vi "2283_calibrarElevador.vi"(0 "input cluster":T2, 1 "Potenciometro linear":dbl(knob) scale=-1.0..1.0) -> (2 "Output elevador":dbl, 3 "Altura":dbl, 4 "Gripp output":bool, 5 "Cuernitos":bool)   [LabVIEW 2014]
uses:
  2283_Outputs autonomo.vi
  <vilib>/addons/control/pid/pid.llb/PID (DBL).vi
  <vilib>/addons/control/pid/NI_PID_pid.lvlib
panel:
  in  "x":dbl=50.0 format="%#_13g"
  in  "PID gains":T1={"proportional gain (Kc)"=0.035, "integral time (Ti, min)"=0.008, "derivative time (Td, min)"=0.0}
  in  "Nivel Cargar":dbl=60.0 format="%#_13g"
  in  "Nivel 1 Caja":dbl=225.0 format="%#_13g"
  in  "Nivel 2 Cajas":dbl=385.0 format="%#_13g"
  in  "Nivel 3 Cajas":dbl=560.0 format="%#_13g"
  in  "Dejar":dbl=530.0 format="%#_13g"
  in  "Nivel Step":dbl=165.0 format="%#_13g"
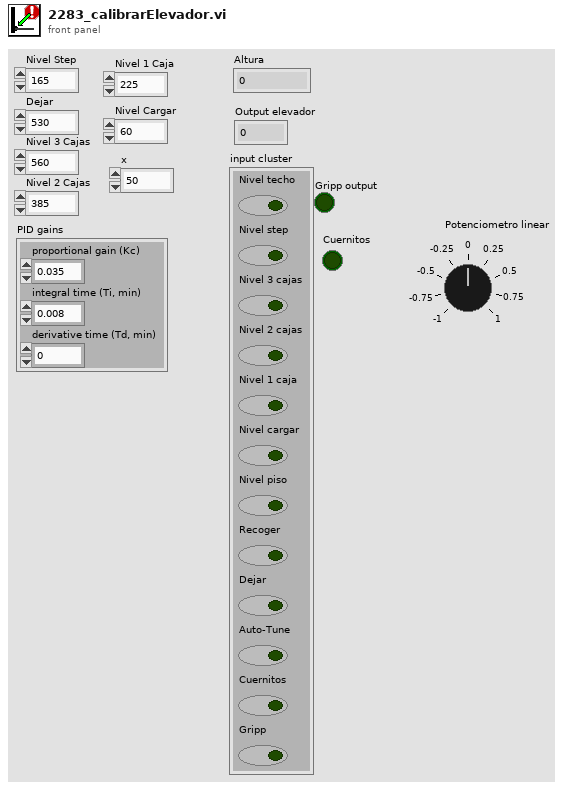
[diagram p1: front panel]
types:
  T1 = cluster{"proportional gain (Kc)":dbl, "integral time (Ti, min)":dbl, "derivative time (Td, min)":dbl}
  T2 = cluster{"Nivel techo":bool, "Nivel step":bool, "Nivel 3 cajas":bool, "Nivel 2 cajas":bool, "Nivel 1 caja":bool, "Nivel cargar":bool, "Nivel piso":bool, "Recoger":bool, "Dejar":bool, "Auto-Tune":bool, "Cuernitos":bool, "Gripp":bool}
  T3 = enum16{"NA", "Nivel cargar", "Nivel Techo", "Nivel step", "Nivel 3 cajas", "Nivel 2 cajas", "Nivel 1 caja", "Nivel Piso"}
  T4 = cluster{"Agarrar caja":bool, "Rotate":dbl, "Dejar caja":bool, "Activar moonwalk":bool, "Alejarse de la caja":bool, "PID LIdar":bool, "Aproach caja":bool, "Comer":bool, "Levante el bote":bool}
  T5 = typedef "WPI_SwitchDevRef.ctl" = cluster{"DevStatus":errorcluster, "DIO Channel":T6, "Controller":T7, "CntIndex":T8, "Normally Closed":bool}
  T6 = typedef "FPGA_DIOChannel.ctl" = enum8{"DIO 0", "DIO 1", "DIO 2", "DIO 3", "DIO 4", "DIO 5", "DIO 6", "DIO 7", "DIO 8", "DIO 9", "DIO MXP 0", "DIO MXP 1", "DIO MXP 2", "DIO MXP 3", "DIO MXP 4", "DIO MXP 5", "DIO MXP 6", "DIO MXP 7", "DIO MXP 8", "DIO MXP 9", "DIO MXP 10", "DIO MXP 11", "DIO MXP 12", "DIO MXP 13", "DIO MXP 14", "DIO MXP 15", "Invalid"}
  T7 = typedef "FPGA_TypedefDigitalModule.ctl" = enum16{"Controller 1"}
  T8 = typedef "FPGA_CounterCtrSystemIndex.ctl" = enum8{"Ctr 0", "Ctr 1", "Ctr 2", "Ctr 3", "Ctr 4", "Ctr 5", "Ctr 6", "Ctr 7", "Invalid"}
  T9 = typedef "WPI_EncoderDevRef.ctl" = cluster{"DevStatus":errorcluster, "EncoderIndex":T10, "CounterIndex":T8, "DistancePerCount":dbl, "Decoding Type":T11}
  T10 = typedef "FPGA_EncoderIdx.ctl" = enum8{"Enc 0", "Enc 1", "Enc 2", "Enc 3", "Enc 4", "Enc 5", "Enc 6", "Enc 7", "Invalid"}
  T11 = typedef "WPI_EncoderType.ctl" = enum16{"1x", "2x", "4x"}
  T12 = cluster{"Nivel techo":dbl, "Nivel 3 cajas":dbl, "Nivel 2 cajas":dbl, "Nivel 1 caja":dbl, "Nivel step":dbl, "Nivel cargar":dbl}
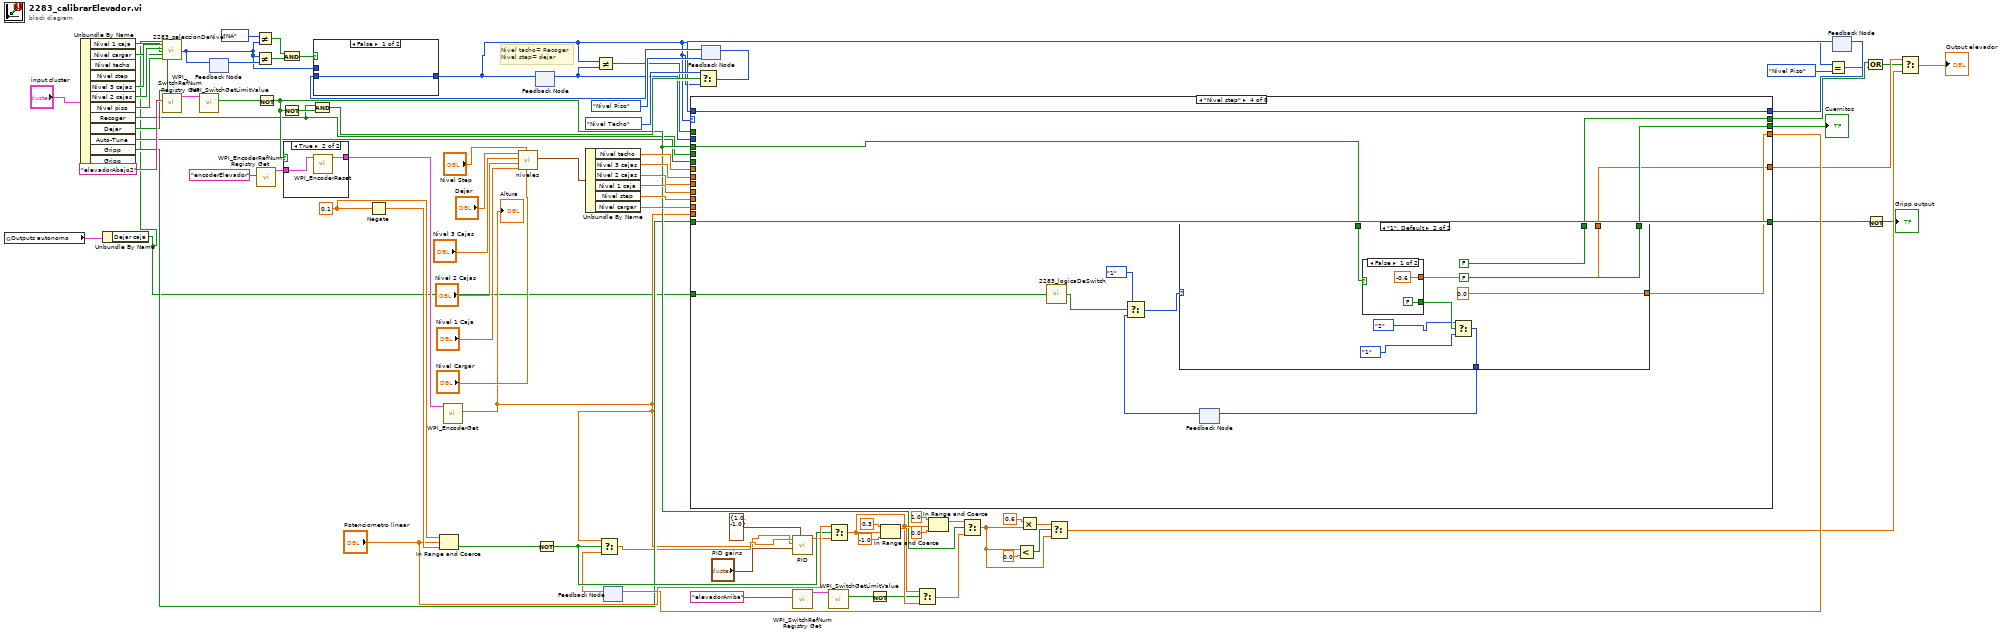
[diagram p0: block diagram]
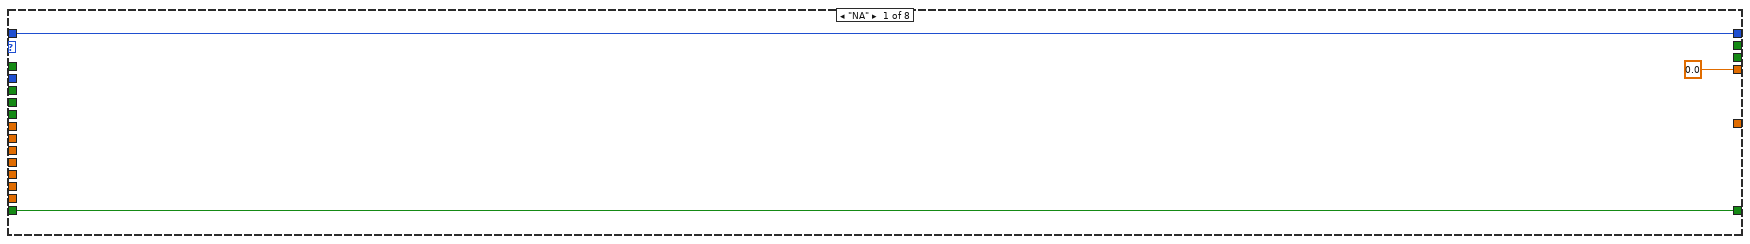
[diagram p2: hidden frame]
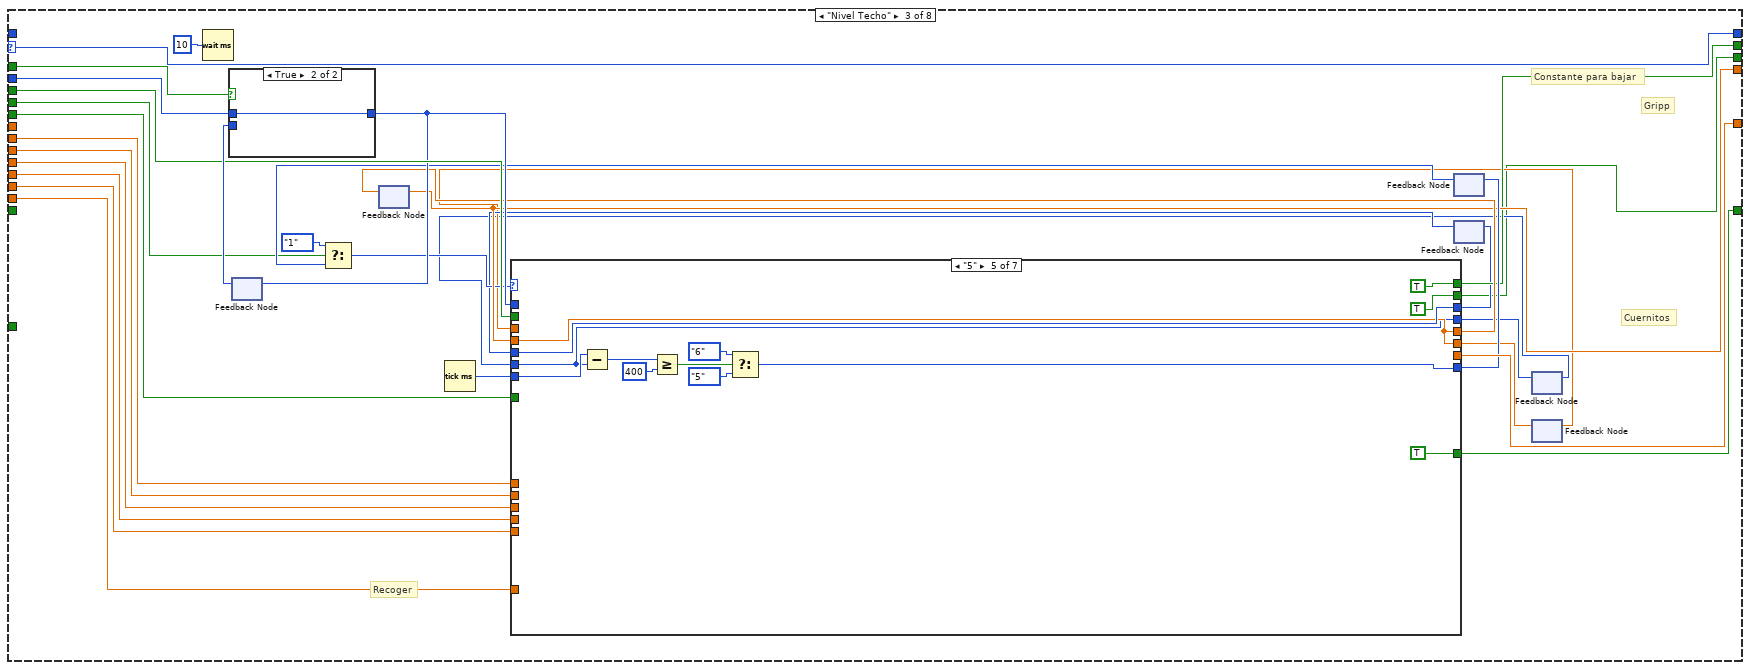
[diagram p4: hidden frame]
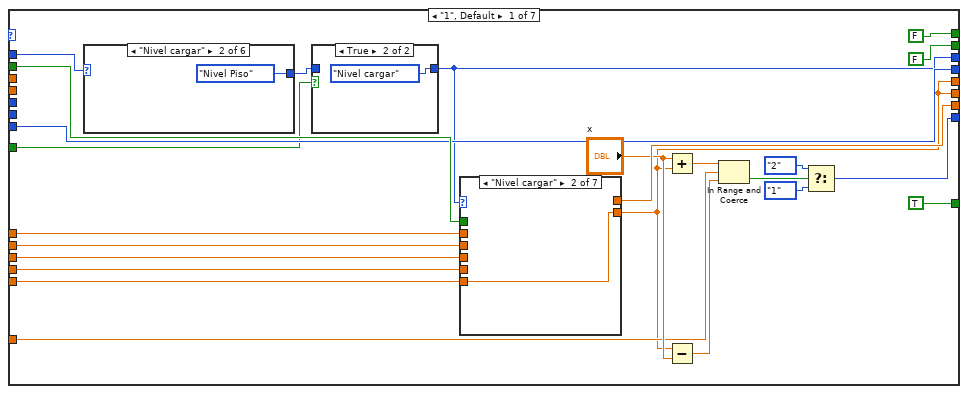
[diagram p5: hidden frame]
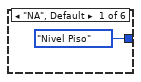
[diagram p7: hidden frame]
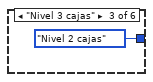
[diagram p8: hidden frame]
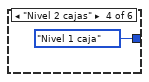
[diagram p9: hidden frame]
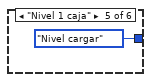
[diagram p10: hidden frame]
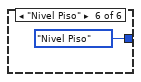
[diagram p11: hidden frame]
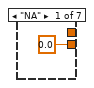
[diagram p12: hidden frame]
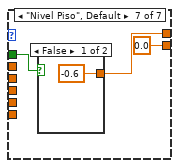
[diagram p17: hidden frame]
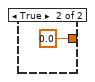
[diagram p18: hidden frame]
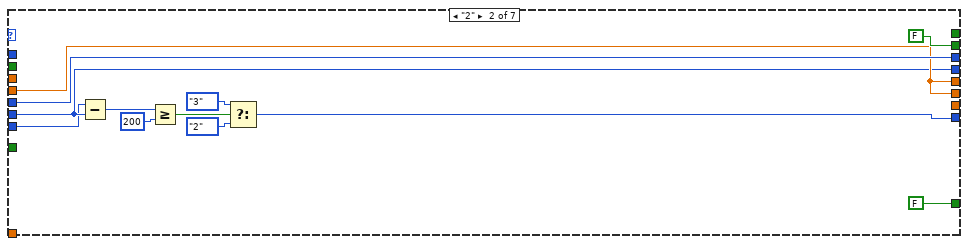
[diagram p19: hidden frame]
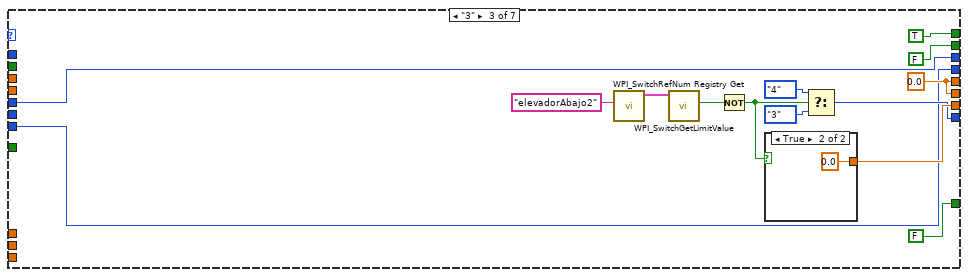
[diagram p20: hidden frame]
diagram:
  w81 = 0.1 ("upper limit")
  # "Nivel techo= Recoger\nNivel step= dejar"
  n1 = global read "2283_Outputs autonomo.vi" "Outputs autonomo"() -> (w2:T4)
  n2 = Unbundle By Name("input cluster") -> ("Nivel 1 caja"=w38:bool, "Nivel cargar"=w39:bool, "Nivel 3 cajas"=w40:bool, "Nivel 2 cajas"=w41:bool, "Nivel piso"=w42:bool, "Recoger"=w10:bool, "Dejar"=w11:bool, "Auto-Tune"=w5:bool, "Gripp"=w15:bool)  [unwired: 3 out]
  n3 = Unbundle By Name(w2) -> ("Dejar caja"=w1:bool)
  n4 = call "2283_seleccionDeNivel.vi"("Cargar"=w1, "Nivel 3 cajas"=w40, "Nivel 2 cajas"=w41, "Nivel 1 caja"=w38, "Nivel cargar"=w39, "Recoger"=w11, "Nivel piso"=w42) -> ("nivel"=w44:T3)  [unwired: 12 in]
  n5 = call <vilib>:"WPI_SwitchRefNum Registry Get.vi"("refnum name"="elevadorAbajo2") -> ("SwitchDevRef"=w83:T5)  [unwired: 9 in, 1 out]
  n6 = call <vilib>:"WPI_SwitchGetLimitValue.vi"("SwitchDevRef"=w83) -> ("Switch Pressed"=w20:bool)  [unwired: 8 in, 2 out]
  n7 = feedback-in #1(w44) -> ()
  n8 = feedback #1() -> (w65:T3)  [unwired: 1 in]
  n9 = Not Equal?(x=T3."NA" ("Enum"), y=w44) -> (x != y?=w66:bool)
  n10 = Not Equal?(x=w44, y=w65) -> (x != y?=w67:bool)
  n11 = call <vilib>:"WPI_EncoderRefNum Registry Get.vi"("refnum name"="encoderElevador") -> ("EncoderDevRef"=w86:T9)  [unwired: 9 in, 1 out]
  n12 = Not(x=w20) -> (.not. x?=w24:bool)
  n13 = And(x=w66, y=w67) -> (x .and. y?=w63:bool)
  n14 = Not(x=w24) -> (.not. x?=w28:bool)
  n15 = case shown="True" w24 {
    tunnel: w86 -> [w89 w91]
    tunnel: [w89 w90] -> w85
    frame False {
    }
    frame True {
      n16 = call <vilib>:"WPI_EncoderReset.vi"("EncoderDevRef"=w91) -> ("EncoderDevRef"=w90:T9)  [unwired: 9 in, 1 out]
    }
  }
  n17 = And(x=w10, y=w28) -> (x .and. y?=w54:bool)
  n18 = Negate(x=w81) -> (-x=w80:dbl)
  n19 = In Range and Coerce(upper limit=w81, x="Potenciometro linear", lower limit=w80) -> (In Range?=w79:bool)  [unwired: 1 out]
  n20 = call <vilib>:"WPI_EncoderGet.vi"("EncoderDevRef"=w85) -> ("Distance"=w3:dbl)  [unwired: 5 in, 5 out]
  "Altura" <- w3
  n21 = call "niveles.vi"("Nivel cargar"="Nivel Cargar", "Nivel step"="Nivel Step", "Nivel 1 caja"="Nivel 1 Caja", "Nivel 2 cajas"="Nivel 2 Cajas", "Nivel 3 cajas"="Nivel 3 Cajas", "Nivel techo"="Dejar") -> ("output cluster"=w51:T12)  [unwired: 5 in]
  n22 = feedback #2() -> (w6:T3)  [unwired: 1 in]
  n23 = Not(x=w79) -> (.not. x?=w77:bool)
  n24 = Unbundle By Name(w51) -> ("Nivel techo"=w60:dbl, "Nivel 3 cajas"=w58:dbl, "Nivel 2 cajas"=w57:dbl, "Nivel 1 caja"=w56:dbl, "Nivel step"=w59:dbl, "Nivel cargar"=w55:dbl)
  n25 = feedback #3() -> (w36:dbl)  [unwired: 1 in]
  n26 = Select(t=w3, s=w77, f=w36) -> (s? t:f=w4:dbl)
  n27 = feedback #4(T3."Nivel Piso" ("Enum")) -> (w62:T3)
  n28 = case shown="False" w63 {
    tunnel: w44 -> [_ w93]
    tunnel: [w92 w93] -> w8
    tunnel: w62 -> [w92 _]
    frame False {
    }
    frame True {
    }
  }
  n29 = feedback-in #2(w8) -> ()
  n30 = Not Equal?(x=w8, y=w6) -> (x != y?=w7:bool)
  n31 = Select(t=T3."Nivel Techo" ("Enum"), s=w54, f=w8) -> (s? t:f=w52:T3)
  n32 = feedback-in #4(w52) -> ()
  n33 = call-poly <vilib>:"PID.vi"("output range"=cluster{"output high":dbl, "output low":dbl} {"output high"=1.0, "output low"=-1.0}, "PID gains"="PID gains", "process variable"=w3, "setpoint"=w4) -> ("output"=w26:dbl)  [unwired: 6 in, 1 out]
  n34 = call <vilib>:"WPI_SwitchRefNum Registry Get.vi"("refnum name"="elevadorArriba") -> ("SwitchDevRef"=w87:T5)  [unwired: 9 in, 1 out]
  n35 = call <vilib>:"WPI_SwitchGetLimitValue.vi"("SwitchDevRef"=w87) -> ("Switch Pressed"=w74:bool)  [unwired: 8 in, 2 out]
  n36 = Select(t="Potenciometro linear", s=w77, f=w26) -> (s? t:f=w68:dbl)
  n37 = Not(x=w74) -> (.not. x?=w29:bool)
  n38 = In Range and Coerce(upper limit=0.3, x=w68, lower limit=-1.0) -> (coerced(x)=w75:dbl)  [unwired: 1 out]
  n39 = Select(t=w75, s=w29, f=w68) -> (s? t:f=w69:dbl)
  n40 = In Range and Coerce(upper limit=1.0, x=w68, lower limit=0.0) -> (coerced(x)=w71:dbl)  [unwired: 1 out]
  n41 = Select(t=w71, s=w24, f=w69) -> (s? t:f=w30:dbl)
  n42 = Less?(x=w30, y=0.0) -> (x < y?=w33:bool)
  n43 = Multiply(x=0.6, y=w30) -> (x*y=w31:dbl)
  n44 = Select(t=w31, s=w33, f=w30) -> (s? t:f=w21:dbl)
  n45 = Equal?(x=w8, y=T3."Nivel Piso" ("Enum")) -> (x = y?=w13:bool)
  n46 = feedback #5() -> (w35:T3)  [unwired: 1 in]
  n47 = case shown="\"Nivel step\"" w8 {
    selector: w8 -> [_ _ w130 _ _ _ _ _]
    tunnel: [0.0 ("upper limit") w99 w117 w287 w312 w315 w318 0.0 ("Nivel 1 caja")] -> w37
    tunnel: w60 -> [_ _ _ _ _ _ _ _]
    tunnel: w59 -> [_ _ w129 _ _ _ _ _]
    tunnel: w58 -> [_ _ w128 _ w312 _ _ _]
    tunnel: w57 -> [_ _ w127 _ _ w315 _ _]
    tunnel: w56 -> [_ _ w126 _ _ _ w318 _]
    tunnel: w55 -> [_ w99 w125 _ _ _ _ _]
    tunnel: [w95 w98 w130 w291 w311 w314 w317 w325] -> w18
    tunnel: w35 -> [w95 w98 _ w291 w311 w314 w317 w325]
    tunnel: w24 -> [_ _ w124 w285 _ _ _ w324]
    tunnel: [_ _ w122 w286 _ _ _ w322] -> w22
    tunnel: w15 -> [w94 w97 _ w290 w310 w313 w316 w321]
    tunnel: [w94 w97 w119 w290 w310 w313 w316 w321] -> w17
    tunnel: w3 -> [_ _ w121 _ _ _ _ _]
    tunnel: [_ _ w101 w288 _ _ _ FALSE] -> w16
    tunnel: [_ _ w113 w289 _ _ _ FALSE] -> w14
    tunnel: w6 -> [_ _ w110 _ _ _ _ _]
    tunnel: w10 -> [_ _ w103 _ _ _ _ _]
    tunnel: w7 -> [_ _ w102 _ _ _ _ _]
    tunnel: w5 -> [_ _ w100 _ _ _ _ _]
    tunnel: w1 -> [_ _ _ w281 _ _ _ _]
    frame "NA" {
    }
    frame "Nivel cargar" {
    }
    frame "Nivel Techo" {
      # "Cuernitos"
      # "Gripp"
      # "Constante para bajar"
      # "Recoger"
      n48 = Wait (ms)(milliseconds to wait=u32 10) -> ()  [unwired: 1 out]
      n49 = feedback #6() -> (w131:T3)  [unwired: 1 in]
      n50 = case shown="True" w102 {
        tunnel: w110 -> [_ w278]
        tunnel: [w277 w278] -> w123
        tunnel: w131 -> [w277 _]
        frame False {
        }
        frame True {
        }
      }
      n51 = feedback-in #6(w123) -> ()
      n52 = feedback #7() -> (w117:dbl)  [unwired: 1 in]
      n53 = Tick Count (ms)() -> (millisecond timer value=w104:u32)
      n54 = feedback #8() -> (w115:enum16{"1", "2", "3", "4", "5", "6", "7"})  [unwired: 1 in]
      n55 = Select(t=enum16{"1", "2", "3", "4", "5", "6", "7"}."1", s=w103, f=w115) -> (s? t:f=w114:enum16{"1", "2", "3", "4", "5", "6", "7"})
      n56 = feedback #9() -> (w111:T3)  [unwired: 1 in]
      n57 = feedback #10() -> (w105:u32)  [unwired: 1 in]
      n58 = feedback #11() -> (w107:dbl)  [unwired: 1 in]
      n59 = case shown="\"5\"" w114 {
        tunnel: w129 -> [w155 _ _ _ _ w248 _]
        tunnel: w128 -> [w154 _ _ _ _ w251 _]
        tunnel: w127 -> [w153 _ _ _ _ w250 _]
        tunnel: w126 -> [w152 _ _ _ _ w249 _]
        tunnel: w125 -> [w151 _ _ _ _ w247 _]
        tunnel: w124 -> [w150 _ _ _ _ w246 _]
        tunnel: w123 -> [w149 _ _ _ _ _ _]
        tunnel: [w132 w183 w189 w212 w227 w234 w275] -> w118
        tunnel: [w148 _ w200 _ _ w245 _] -> w122
        tunnel: w121 -> [w145 _ _ _ _ w235 _]
        tunnel: [w140 w181 w197 w209 w224 w236 enum16{"1", "2", "3", "4", "5", "6", "7"}."7"] -> w120
        tunnel: [TRUE FALSE FALSE TRUE TRUE TRUE TRUE] -> w119
        tunnel: w117 -> [_ w183 _ w212 w227 _ _]
        tunnel: [FALSE ("Cuernitos") FALSE ("Cuernitos") FALSE ("Cuernitos") FALSE ("Cuernitos") TRUE ("Cuernitos") FALSE ("Cuernitos") FALSE ("Cuernitos")] -> w101
        tunnel: [FALSE _ TRUE TRUE TRUE _ _] -> w113
        tunnel: [w134 w184 w190 w213 w228 w243 w273] -> w112
        tunnel: w111 -> [_ w184 w190 w213 w228 w243 w273]
        tunnel: [w132 w183 w189 w212 w227 w234 w275] -> w108
        tunnel: w107 -> [_ _ _ _ _ _ w275]
        tunnel: [w136 w176 w188 w204 w218 w233 w272] -> w106
        tunnel: w105 -> [_ w176 _ w204 w218 _ _]
        tunnel: w104 -> [w136 w175 w188 w205 w220 w233 w272]
        tunnel: w100 -> [w133 _ _ _ _ w229 _]
        frame "1", Default {
          n60 = case shown="\"Nivel cargar\"" w149 {
            tunnel: [T3."Nivel Piso" ("Enum") T3."Nivel Piso" ("Enum") T3."Nivel 2 cajas" ("Enum") T3."Nivel 1 caja" ("Enum") T3."Nivel cargar" ("Enum") T3."Nivel Piso" ("Enum")] -> w135
            frame "NA", Default {
            }
            frame "Nivel cargar" {
            }
            frame "Nivel 3 cajas" {
            }
            frame "Nivel 2 cajas" {
            }
            frame "Nivel 1 caja" {
            }
            frame "Nivel Piso" {
            }
          }
          n61 = case shown="True" w133 {
            tunnel: w135 -> [w156 _]
            tunnel: [w156 T3."Nivel cargar" ("Enum")] -> w134
            frame False {
            }
            frame True {
            }
          }
          n62 = case shown="\"Nivel cargar\"" w134 {
            tunnel: [0.0 ("upper limit") w165 w166 w167 w168 w169 0.0 ("Nivel 1 caja")] -> w132
            tunnel: w155 -> [_ _ w166 _ _ _ _]
            tunnel: w154 -> [_ _ _ w167 _ _ _]
            tunnel: w153 -> [_ _ _ _ w168 _ _]
            tunnel: w152 -> [_ _ _ _ _ w169 _]
            tunnel: w151 -> [_ w165 _ _ _ _ _]
            tunnel: w150 -> [_ _ _ _ _ _ w172]
            tunnel: [_ _ _ _ _ _ w170] -> w148
            frame "NA" {
            }
            frame "Nivel cargar" {
            }
            frame "Nivel step" {
            }
            frame "Nivel 3 cajas" {
            }
            frame "Nivel 2 cajas" {
            }
            frame "Nivel 1 caja" {
            }
            frame "Nivel Piso", Default {
              n63 = case shown="False" w172 {
                tunnel: [-0.6 ("upper limit") 0.0 ("upper limit")] -> w170
                frame False {
                }
                frame True {
                }
              }
            }
          }
          n64 = Add(x="x", y=w132) -> (x+y=w144:dbl)
          n65 = Subtract(x=w132, y="x") -> (x-y=w147:dbl)
          n66 = In Range and Coerce(upper limit=w144, x=w145, lower limit=w147) -> (In Range?=w143:bool)  [unwired: 1 out]
          n67 = Select(t=enum16{"1", "2", "3", "4", "5", "6", "7"}."2", s=w143, f=enum16{"1", "2", "3", "4", "5", "6", "7"}."1") -> (s? t:f=w140:enum16{"1", "2", "3", "4", "5", "6", "7"})
        }
        frame "2" {
          n68 = Subtract(x=w175, y=w176) -> (x-y=w179:u32)
          n69 = Greater Or Equal?(x=w179, y=u32 200) -> (x >= y?=w177:bool)
          n70 = Select(t=enum16{"1", "2", "3", "4", "5", "6", "7"}."3", s=w177, f=enum16{"1", "2", "3", "4", "5", "6", "7"}."2") -> (s? t:f=w181:enum16{"1", "2", "3", "4", "5", "6", "7"})
        }
        frame "3" {
          w189 = 0.0 ("Nivel 1 caja")
          n71 = call <vilib>:"WPI_SwitchRefNum Registry Get.vi"("refnum name"="elevadorAbajo2") -> ("SwitchDevRef"=w194:T5)  [unwired: 9 in, 1 out]
          n72 = call <vilib>:"WPI_SwitchGetLimitValue.vi"("SwitchDevRef"=w194) -> ("Switch Pressed"=w193:bool)  [unwired: 8 in, 2 out]
          n73 = Not(x=w193) -> (.not. x?=w187:bool)
          n74 = case shown="True" w187 {
            tunnel: [-0.6 ("upper limit") 0.0 ("upper limit")] -> w200
            frame False {
            }
            frame True {
            }
          }
          n75 = Select(t=enum16{"1", "2", "3", "4", "5", "6", "7"}."4", s=w187, f=enum16{"1", "2", "3", "4", "5", "6", "7"}."3") -> (s? t:f=w197:enum16{"1", "2", "3", "4", "5", "6", "7"})
        }
        frame "4" {
          n76 = Subtract(x=w205, y=w204) -> (x-y=w208:u32)
          n77 = Greater Or Equal?(x=w208, y=u32 200) -> (x >= y?=w206:bool)
          n78 = Select(t=enum16{"1", "2", "3", "4", "5", "6", "7"}."5", s=w206, f=enum16{"1", "2", "3", "4", "5", "6", "7"}."4") -> (s? t:f=w209:enum16{"1", "2", "3", "4", "5", "6", "7"})
        }
        frame "5" {
          n79 = Subtract(x=w220, y=w218) -> (x-y=w222:u32)
          n80 = Greater Or Equal?(x=w222, y=u32 400) -> (x >= y?=w219:bool)
          n81 = Select(t=enum16{"1", "2", "3", "4", "5", "6", "7"}."6", s=w219, f=enum16{"1", "2", "3", "4", "5", "6", "7"}."5") -> (s? t:f=w224:enum16{"1", "2", "3", "4", "5", "6", "7"})
        }
        frame "6" {
          w241 = 2.0 ("x")
          n82 = case shown="\"Nivel 3 cajas\"" w243 {
            tunnel: [T3."Nivel cargar" ("Enum") T3."Nivel 1 caja" ("Enum") T3."Nivel 3 cajas" ("Enum") T3."Nivel 3 cajas" ("Enum") T3."Nivel 2 cajas" ("Enum") T3."Nivel cargar" ("Enum")] -> w231
            frame "NA", Default {
            }
            frame "Nivel cargar" {
            }
            frame "Nivel 3 cajas" {
            }
            frame "Nivel 2 cajas" {
            }
            frame "Nivel 1 caja" {
            }
            frame "Nivel Piso" {
            }
          }
          n83 = case shown="True" w229 {
            tunnel: w231 -> [w252 _]
            tunnel: [w252 T3."Nivel 2 cajas" ("Enum")] -> w230
            frame False {
            }
            frame True {
            }
          }
          n84 = case shown="\"Nivel 3 cajas\"" w230 {
            tunnel: [0.0 ("upper limit") w261 w262 w263 w264 w265 0.0 ("Nivel 1 caja")] -> w234
            tunnel: w248 -> [_ _ w262 _ _ _ _]
            tunnel: w251 -> [_ _ _ w263 _ _ _]
            tunnel: w250 -> [_ _ _ _ w264 _ _]
            tunnel: w249 -> [_ _ _ _ _ w265 _]
            tunnel: w247 -> [_ w261 _ _ _ _ _]
            tunnel: w246 -> [_ _ _ _ _ _ w268]
            tunnel: [_ _ _ _ _ _ w266] -> w245
            frame "NA" {
            }
            frame "Nivel cargar" {
            }
            frame "Nivel step" {
            }
            frame "Nivel 3 cajas" {
            }
            frame "Nivel 2 cajas" {
            }
            frame "Nivel 1 caja" {
            }
            frame "Nivel Piso", Default {
              n85 = case shown="False" w268 {
                tunnel: [-0.6 ("upper limit") 0.0 ("upper limit")] -> w266
                frame False {
                }
                frame True {
                }
              }
            }
          }
          n86 = Add(x=w241, y=w234) -> (x+y=w240:dbl)
          n87 = Subtract(x=w234, y=w241) -> (x-y=w242:dbl)
          n88 = In Range and Coerce(upper limit=w240, x=w235, lower limit=w242) -> (In Range?=w239:bool)  [unwired: 1 out]
          n89 = Select(t=enum16{"1", "2", "3", "4", "5", "6", "7"}."7", s=w239, f=enum16{"1", "2", "3", "4", "5", "6", "7"}."6") -> (s? t:f=w236:enum16{"1", "2", "3", "4", "5", "6", "7"})
        }
        frame "7" {
        }
      }
      n90 = feedback-in #7(w118) -> ()
      n91 = feedback-in #8(w120) -> ()
      n92 = feedback-in #9(w112) -> ()
      n93 = feedback-in #10(w106) -> ()
      n94 = feedback-in #11(w108) -> ()
    }
    frame "Nivel step" {
      n95 = call "2283_logicaDeSwitch.vi"("Input"=w281) -> ("Output"=w280:bool)
      n96 = feedback #12() -> (w283:enum16{"2", "1"})  [unwired: 1 in]
      n97 = Select(t=enum16{"2", "1"}."1", s=w280, f=w283) -> (s? t:f=w282:enum16{"2", "1"})
      n98 = case shown="\"1\", Default" w282 {
        selector: w282 -> [w296 _]
        tunnel: [FALSE FALSE] -> w289
        tunnel: [FALSE FALSE] -> w288
        tunnel: [0.0 ("Nivel 1 caja") 0.0 ("Nivel 1 caja")] -> w287
        tunnel: [0.0 ("upper limit") w302] -> w286
        tunnel: w285 -> [_ w301]
        tunnel: [w296 w299] -> w284
        frame "2" {
        }
        frame "1", Default {
          n99 = case shown="False" w301 {
            tunnel: [-0.6 ("upper limit") 0.0 ("upper limit")] -> w302
            tunnel: [FALSE TRUE] -> w300
            frame False {
            }
            frame True {
            }
          }
          n100 = Select(t=enum16{"2", "1"}."2", s=w300, f=enum16{"2", "1"}."1") -> (s? t:f=w299:enum16{"2", "1"})
        }
      }
      n101 = feedback-in #12(w284) -> ()
    }
    frame "Nivel 3 cajas" {
    }
    frame "Nivel 2 cajas" {
    }
    frame "Nivel 1 caja" {
    }
    frame "Nivel Piso", Default {
      (unwired) T3."Nivel Piso" ("Enum")
      n102 = case shown="False" w324 {
        tunnel: [-0.6 ("upper limit") 0.0 ("upper limit")] -> w322
        frame False {
        }
        frame True {
        }
      }
    }
  }
  "Cuernitos" <- w16
  n103 = feedback-in #3(w37) -> ()
  n104 = feedback-in #5(w18) -> ()
  n105 = Or(x=w14, y=w13) -> (x .or. y?=w12:bool)
  n106 = Not(x=w17) -> (.not. x?=→"Gripp output":bool)
  n107 = Select(t=w22, s=w12, f=w21) -> (s? t:f=→"Output elevador":dbl)
